vi "Get Name.vi"(11 "File Provider in":refnum<class "File Provider.lvclass">) -> (2 "Name":string, 3 "File Provider out":refnum<class "File Provider.lvclass">)   [LabVIEW 2024, in "File Provider.lvlib" / "File Provider.lvclass"]
uses:
  File Provider.lvclass
  File Provider.lvclass/File Provider.ctl
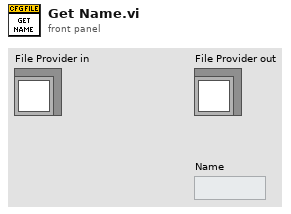
[diagram p1: front panel]
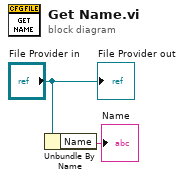
[diagram p0: block diagram]
diagram:
  n1 = Unbundle By Name("File Provider in") -> ("Name"=→"Name":string)
  "File Provider out" <- "File Provider in"
